vi "Event Nested.vi"(8 "Alias":string, 10 "Msg":refnum<class "Msg.lvclass">, 11 "Base Queue Actor in":refnum<class "Base Queue Actor.lvclass">) -> (3 "Base Queue Actor out":refnum<class "Base Queue Actor.lvclass">)   [LabVIEW 2021, in "jettl.lvlib" / "Base Queue Actor.lvclass"]
uses:
  Base Queue Actor.lvclass
  Msg/Msg/Msg.lvclass
  Base Queue Actor.lvclass/Base Queue Actor.ctl
  jettl.lvlib
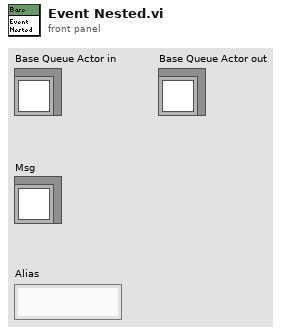
[diagram p1: front panel]
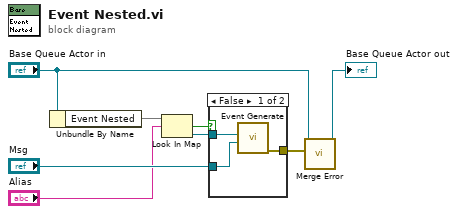
[diagram p0: block diagram]
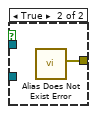
[diagram p2: hidden frame]
diagram:
  n1 = Unbundle By Name("Base Queue Actor in") -> ("Event Nested"=w7:map{string, refnum<data-value>})
  n2 = Look In Map(map=w7, key="Alias") -> (key not found?=w6:bool, value=w8:refnum<data-value>)  [unwired: 1 in]
  n3 = case shown="False" w6 {
    tunnel: [w9 w12] -> w5
    tunnel: "Msg" -> [w10 _]
    tunnel: w8 -> [w11 _]
    frame False {
      n4 = call "Event Generate.vi"("Msg"=w10, "Event"=w11) -> ("error out"=w9:errorcluster)  [unwired: 9 in]
    }
    frame True {
      n5 = call "Alias Does Not Exist Error.vi"() -> ("Error"=w12:errorcluster)  [unwired: 11 in]
    }
  }
  n6 = call-dynamic "Merge Error.vi"("Error"=w5, "Base Queue Actor in"="Base Queue Actor in") -> ("Base Queue Actor out"=→"Base Queue Actor out":refnum<class "Base Queue Actor.lvclass">)  [unwired: 9 in]
